vi "displayControlElement2.vi"(10 "viewThisComponent":refnum<class "ViewThisComponent.lvclass">) -> ()   [LabVIEW 2016, in "sedSpectrometerViewElements.lvlib"]
doc: "Displays a control element."
uses:
  sedSpectrometerViewElements.lvlib
  ViewThisComponent/ViewThisComponent.lvclass
  home/harini/tcs/ts_FiberSpectrograph/ComponentTemplateCore/ComponentModel/ComponentModel/View/View.lvclass
  ts_sallv_FiberSpectrograph/DataTypes/logevent_detailedState.ctl
  Typedefs/SubDataSignal.ctl
  Typedefs/FiberSpectrographTypedefs.lvlib
  ComponentTemplateCore/ComponentModel/ComponentModel/View/View.lvclass
  ts_sallv_FiberSpectrograph/SALLV_FiberSpectrograph.lvlib
panel:
  in  "sendAValueIsTrue":bool caption="Start"
  in  "aValue":dbl[unit] format="%.2f"
  in  "DoThisIsTrue":bool caption="Start"
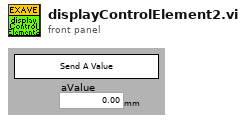
[diagram p1: front panel]
types:
  T1 = typedef "TypedefsDataEvents.lvlib/PubDataEvents.ctl" = cluster{"AppliedSettingsMatchStart":refnum<user-event>, "SettingVersions":refnum<user-event>, "SummaryState":refnum<user-event>, "RejectedCommand":refnum<user-event>, "DetailedState":refnum<user-event>, "ErrorCode":refnum<user-event>, "Heartbeat":refnum<user-event>, "LoopTime_ms":refnum<user-event>, "LoopTimeOutOfRange":refnum<user-event>, "Timestamp":refnum<user-event>, "TimeOut":refnum<user-event>, "MeasuredSpectrum":refnum<user-event>, "LargeFileObjectAvailable":refnum<user-event>}
  T2 = typedef "SALLV_FiberSpectrograph.lvlib/logevent_detailedState.ctl" = cluster{"detailedState":i32, "priority":i32}
  T3 = typedef "FiberSpectrographTypedefs.lvlib/SubDataSignal.ctl" = enum16{"disable", "enable", "exit", "standby", "HeartbeatIn", "start", "captureSpectImage"}
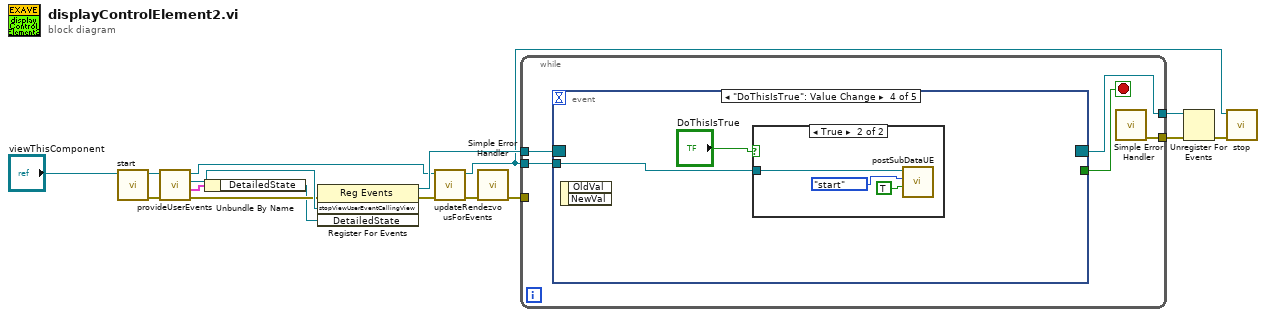
[diagram p0: block diagram]
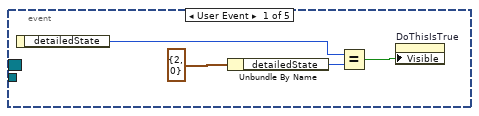
[diagram p2: hidden frame]
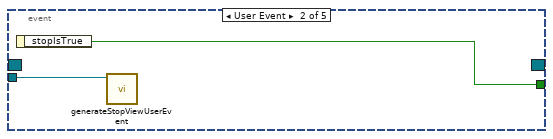
[diagram p3: hidden frame]
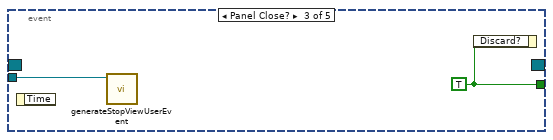
[diagram p4: hidden frame]
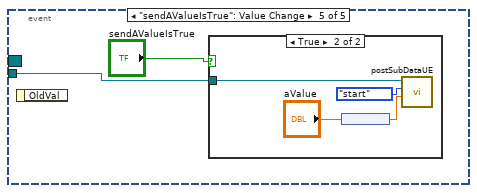
[diagram p6: hidden frame]
diagram:
  n1 = call-dynamic "start.vi"("View in"="viewThisComponent") -> ("error out"=w7:errorcluster, "View out"=w12:refnum<class "ViewThisComponent.lvclass">)  [unwired: 9 in]
  n2 = call "provideUserEvents.vi"("error in (no error)"=w7, "ViewThisComponent in"=w12) -> ("error out"=w13:errorcluster, "pubDataEvents"=w14:T1, "stopViewUserEventCallingView"=w15:refnum<user-event>, "ViewThisComponent out"=w2:refnum<class "ViewThisComponent.lvclass">)  [unwired: 6 in]
  n3 = Unbundle By Name(w14) -> ("DetailedState"=w10:refnum<user-event>)
  n4 = register-events(error in=w13, w15, w10) -> (reference out=w11:refnum<event-registration>, error out=w4:errorcluster)  [unwired: 1 in]
  n5 = call "updateRendezvousForEvents.vi"("error in (no error)"=w4, "View in"=w2) -> ("error out"=w3:errorcluster, "View out"=w1:refnum<class "ViewThisComponent.lvclass">)  [unwired: 8 in]
  n6 = call <vilib>:"Simple Error Handler.vi"("error in (no error)"=w3) -> ("error out"=w5:errorcluster)  [unwired: 4 in, 4 out]
  n7 = while {
    tunnel: w11 -> [w21]
    tunnel: w1 -> [w20]
    tunnel: [w19] -> w6
    tunnel: [w17] -> w9
    tunnel: w5 -> [_]
    stop <- w18 stop-if-true
    n8 = event shown="[3] \"DoThisIsTrue\": Value Change" {
      selector: w21 -> [_ _ _ _ _]
      dyn-events: [_ _ _ _ _] -> w17
      timeout: _ -> [_ _ _ _ _]
      tunnel: w20 -> [_ w26 w29 w30 w35]
      tunnel: [_ w27 w28 _ _] -> w18
      event User Event {
        n9 = event-data() -> ("detailedState"=w24:i32)  [unwired: 1 in]
        n10 = Unbundle By Name(T2 {"detailedState"=2, "priority"=0} ("logevent_DetailedState")) -> ("detailedState"=w22:i32)
        n11 = Equal?(x=w24, y=w22) -> (x = y?=w25:bool)
        n12 = property on="DoThisIsTrue" class="Bool"("Visible"=w25) -> ()  [unwired: 2 in, 2 out]
      }
      event User Event {
        n13 = event-data() -> ("stopIsTrue"=w27:bool)  [unwired: 1 in]
        n14 = call "generateStopViewUserEvent.vi"("View in"=w26) -> ()  [unwired: 9 in, 2 out]
      }
      event Panel Close? {
        w28 = TRUE ("Discard?")
        n15 = event-data() -> ()  [unwired: 1 in, 1 out]
        n16 = call "generateStopViewUserEvent.vi"("View in"=w29) -> ()  [unwired: 9 in, 2 out]
        n17 = event-data("Discard?"=w28) -> ()  [unwired: 1 in, 1 out]
      }
      event "DoThisIsTrue": Value Change {
        n18 = event-data() -> ()  [unwired: 1 in, 2 out]
        n19 = case shown="True" "DoThisIsTrue" {
          tunnel: w30 -> [_ w32]
          frame False {
          }
          frame True {
            n20 = call "postSubDataUE.vi"("value"=TRUE ("Start"), "subDataSV"=SubDataSignal."start" ("SubDataSV"), "ViewThisComponent in"=w32) -> ()  [unwired: 7 in, 2 out]
          }
        }
      }
      event "sendAValueIsTrue": Value Change {
        n21 = event-data() -> ()  [unwired: 1 in, 1 out]
        n22 = case shown="True" "sendAValueIsTrue" {
          tunnel: w35 -> [_ w37]
          frame False {
          }
          frame True {
            n23 = node("aValue") -> (w38:dbl)
            n24 = call "postSubDataUE.vi"("value"=w38, "subDataSV"=SubDataSignal."start" ("SubDataSV"), "ViewThisComponent in"=w37) -> ()  [unwired: 7 in, 2 out]
          }
        }
      }
    }
    n25 = call <vilib>:"Simple Error Handler.vi"() -> ("error out"=w19:errorcluster)  [unwired: 5 in, 4 out]
  }
  n26 = Unregister For Events(event registration refnum=w9, error in=w6) -> (error out=w8:errorcluster)
  n27 = call-dynamic "stop.vi"("error in (no error)"=w8, "View in"=w1) -> ()  [unwired: 8 in, 2 out]
